vi "ConfigureMeasure.vi"(7 "SMU":T1, 8 "Error In":errorcluster, 10 "Measure Configuration":T2={"Enabled?"=FALSE, "Count"=1, "Interval (sec)"=0.025, "Voltage Auto Range Enabled?"=TRUE, "Voltage High Limit (V or A)"=0.0, "Voltage Low Limit (V or A)"=0.0, "Current Auto Range Enabled?"=TRUE, "Current High Limit (V or A)"=0.0, "Current Low Limit (V or A)"=0.0} {"Count" min=1 step=1}, 11 "Keithley 2602 In":refnum<visa-resource-name>) -> (0 "Error Out":errorcluster, 3 "Keithley 2602 Out":refnum<visa-resource-name>)   [LabVIEW 2013]
uses:
  MeasureConfiguration.ctl
  driver/Public/Controls/SMU.ctl
  driver/Public/Controls/RangeFunction.ctl
  driver/Keithley-2602.lvlib
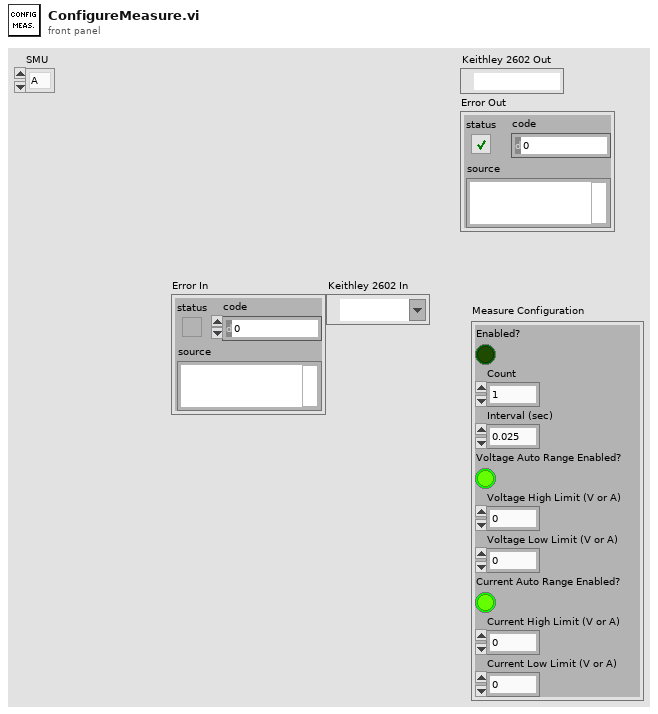
[diagram p1: front panel]
types:
  T1 = typedef "Keithley-2602.lvlib/SMU.ctl" = enum16{"A", "B"}
  T2 = typedef "MeasureConfiguration.ctl" = cluster{"Enabled?":bool, "Count":u8, "Interval (sec)":dbl, "Voltage Auto Range Enabled?":bool, "Voltage High Limit (V or A)":dbl, "Voltage Low Limit (V or A)":dbl, "Current Auto Range Enabled?":bool, "Current High Limit (V or A)":dbl, "Current Low Limit (V or A)":dbl}
  T3 = typedef "Keithley-2602.lvlib/RangeFunction.ctl" = enum16{"Voltage", "Current"}
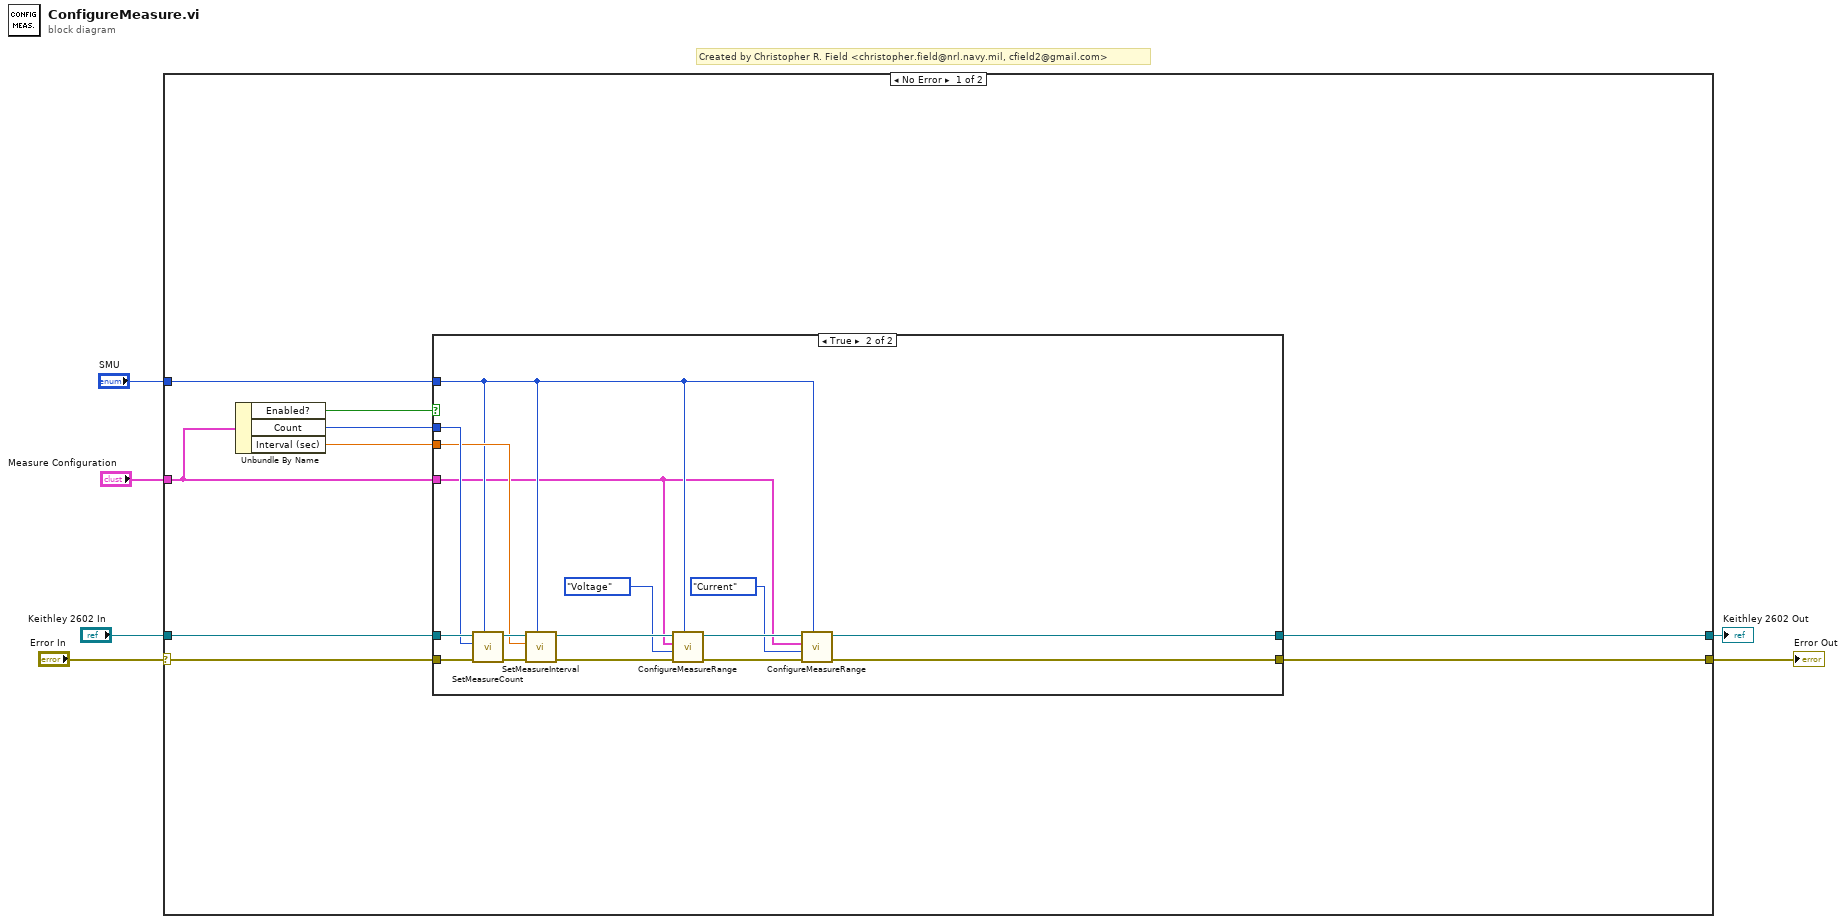
[diagram p0: block diagram]
diagram:
  # "Created by Christopher R. Field <christopher.field@nrl.navy.mil, cfield2@gmail.com>"
  n1 = case shown="No Error" "Error In" {
    selector: "Error In" -> [w14 w34]
    tunnel: "Measure Configuration" -> [w7 _]
    tunnel: "Keithley 2602 In" -> [w15 w35]
    tunnel: "SMU" -> [w10 _]
    tunnel: [w9 w35] -> w2
    tunnel: [w8 w34] -> w1
    frame No Error {
      n2 = Unbundle By Name(w7) -> ("Enabled?"=w13:bool, "Count"=w12:u8, "Interval (sec)"=w11:dbl)
      n3 = case shown="True" w13 {
        tunnel: w15 -> [w17 w31]
        tunnel: w14 -> [w16 w30]
        tunnel: w12 -> [_ w29]
        tunnel: w10 -> [_ w23]
        tunnel: w11 -> [_ w28]
        tunnel: [w17 w19] -> w9
        tunnel: [w16 w18] -> w8
        tunnel: w7 -> [_ w21]
        frame False {
        }
        frame True {
          n4 = call "SetMeasureCount.vi"("SMU"=w23, "Error In"=w30, "Count"=w29, "Keithley 2602 In"=w31) -> ("Error Out"=w32:errorcluster, "Keithley 2602 Out"=w33:refnum<visa-resource-name>)  [unwired: 6 in]
          n5 = call "SetMeasureInterval.vi"("SMU"=w23, "Error In"=w32, "Interval"=w28, "Keithley 2602 In"=w33) -> ("Error Out"=w25:errorcluster, "Keithley 2602 Out"=w27:refnum<visa-resource-name>)  [unwired: 6 in]
          n6 = call "ConfigureMeasureRange.vi"("SMU"=w23, "Error In"=w25, "Range Function"=RangeFunction."Voltage", "Measure Configuration"=w21, "Keithley 2602 In"=w27) -> ("Error Out"=w22:errorcluster, "Keithley 2602 Out"=w24:refnum<visa-resource-name>)  [unwired: 5 in]
          n7 = call "ConfigureMeasureRange.vi"("SMU"=w23, "Error In"=w22, "Range Function"=RangeFunction."Current", "Measure Configuration"=w21, "Keithley 2602 In"=w24) -> ("Error Out"=w18:errorcluster, "Keithley 2602 Out"=w19:refnum<visa-resource-name>)  [unwired: 5 in]
        }
      }
    }
    frame Error {
    }
  }
  "Keithley 2602 Out" <- w2
  "Error Out" <- w1
